vi "Test Pass if String Input Matches.vi"(8 "error in (no error)":errorcluster, 11 "Test Case In":refnum<class "Argument Comparison Test.lvclass">) -> (0 "error out":errorcluster, 3 "Test Case Out":refnum<class "Argument Comparison Test.lvclass">)   [LabVIEW 2020, in "Argument Comparison Test.lvclass"]
uses:
  Argument Comparison Test/Argument Comparison Test.lvclass
  C:/Program Files (x86)/National Instruments/LabVIEW 2020/vi.lib/Astemes/LUnit/Test Case.lvclass
  Test Doubles/Test Interface Responsive Mock/Test Interface Mock.lvclass
  C:/git/astemes-lmock/source/Framework/Mock/Mock.lvclass
  Argument Comparison Test/Argument Comparison Test.lvclass/Argument Comparison Test.ctl
  Expectation Test/Responsive Mock Expectation Test.lvclass
  source/Expectations/One/One.lvclass
  C:/git/astemes-lmock/tests/Test Doubles/Test Interface Responsive Mock/Test Interface Mock.lvclass
  C:/git/astemes-lmock/tests/Test Doubles/Test Interface/Test Interface.lvclass
  C:/git/astemes-lmock/tests/Expectation Test/Responsive Mock Expectation Test.lvclass
  C:/Program Files (x86)/National Instruments/LabVIEW 2020/vi.lib/Astemes/LUnit/LUnit Runnable.lvclass
  C:/git/astemes-lmock/tests/Argument Comparison Test/Argument Comparison Test.lvclass
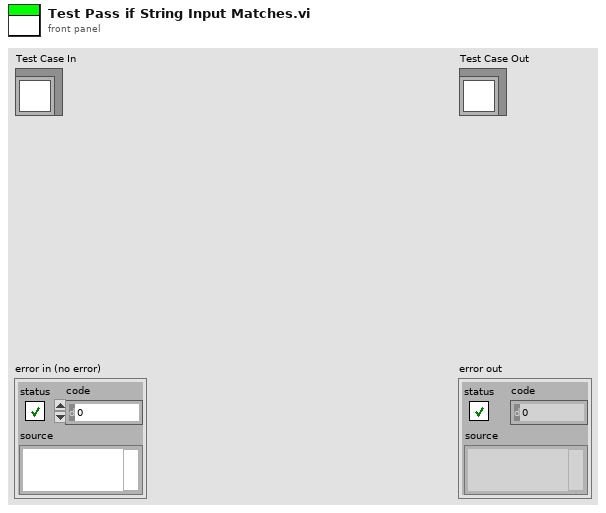
[diagram p1: front panel]
types:
  T1 = enum16{"", "Passed", "Failed", "Error", "Skipped", "Setup Error", "Broken", "Teardown Error"}
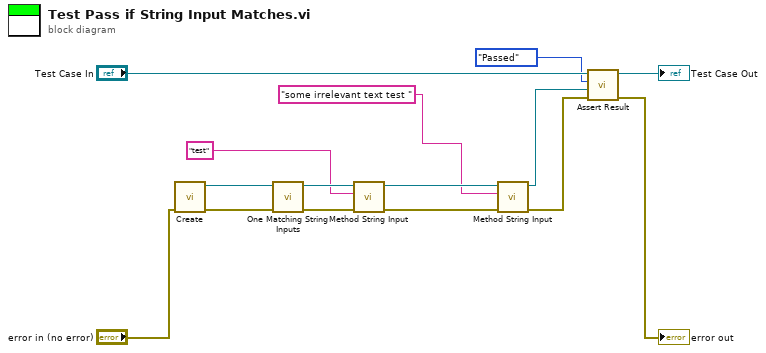
[diagram p0: block diagram]
diagram:
  n1 = call "Create.vi"("error in (no error)"="error in (no error)") -> ("error out"=w14:errorcluster, "Test Interface Mock Out"=w15:refnum<class "Test Interface Mock.lvclass">)  [unwired: 9 in]
  n2 = call "One Matching String Inputs.vi"("error in (no error)"=w14, "Mock in"=w15) -> ("error out"=w12:errorcluster, "Mock out"=w13:refnum<class "Test Interface Mock.lvclass">)  [unwired: 8 in]
  n3 = call-dynamic "Method String Input.vi"("error in (no error)"=w12, "String Input"="test", "Test Interface Mock In"=w13) -> ("error out"=w11:errorcluster, "Test Interface Mock Out"=w5:refnum<class "Test Interface Mock.lvclass">)  [unwired: 7 in]
  n4 = call-dynamic "Method String Input.vi"("error in (no error)"=w11, "String Input"="some irrelevant text test ", "Test Interface Mock In"=w5) -> ("error out"=w4:errorcluster, "Test Interface Mock Out"=w3:refnum<class "Test Interface Mock.lvclass">)  [unwired: 7 in]
  n5 = call "Assert Result.vi"("error in (no error)"=w4, "Mock"=w3, "Status"=T1."Passed", "LUnit Test Case In"="Test Case In") -> ("error out"=→"error out":errorcluster, "LUnit Test Case Out"=→"Test Case Out":refnum<class "Argument Comparison Test.lvclass">)  [unwired: 6 in]
